vi "4155C Output-FPP Config SMUs v3.1.vi"(0 "VISA resource name in":refnum<visa-resource-name>, 1 "Pulse period":dbl=0.005 min=0.005 max=1.0 step=0.0001 format="%.4f", 2 "FPP - Source":u32(ring)=6 items=["SMU1  ", "SMU2  ", "SMU3  ", "SMU4  ", "SMU5  ", "SMU6  ", "VSU1  ", "VSU2  "], 3 "Pulse width":dbl=0.0005 min=0.0005 max=0.1 step=0.0001 format="%.4f", 4 "Base voltage":dbl format="%^.4e", 5 "error in (no error)":errorcluster, 6 "sweep method":u16(ring) items=["Continuous", "Pulsed"], 7 "FPP - Gate":u32(ring)=2 items=["SMU1  ", "SMU2  ", "SMU3  ", "SMU4  ", "SMU5  ", "SMU6  ", "VSU1  ", "VSU2  "], 8 "FPP - Drain":u32(ring)=1 items=["SMU1  ", "SMU2  ", "SMU3  ", "SMU4  ", "SMU5  ", "SMU6  ", "VSU1  ", "VSU2  "], 9 "FPP - Probe 1":u32(ring) items=["SMU1  ", "SMU2  ", "SMU3  ", "SMU4  ", "SMU5  ", "SMU6  ", "VSU1  ", "VSU2  "], 10 "Gate mode":u16(ring) items=["Auto", "Limited", "Fixed"], 11 "Source/drain mode":u16(ring) items=["Auto", "Limited", "Fixed"], 12 "Gate Range":u8(slide)=6 max=11 scale=0.0..11.0, 13 "Source/drain Range":u8(slide)=6 max=11 scale=0.0..11.0, 15 "FPP - Probe 2":u32(ring)=3 items=["SMU1  ", "SMU2  ", "SMU3  ", "SMU4  ", "SMU5  ", "SMU6  ", "VSU1  ", "VSU2  "]) -> (14 "VISA Resource Name out":refnum<visa-resource-name>, 19 "error out":errorcluster)   [LabVIEW 2016]
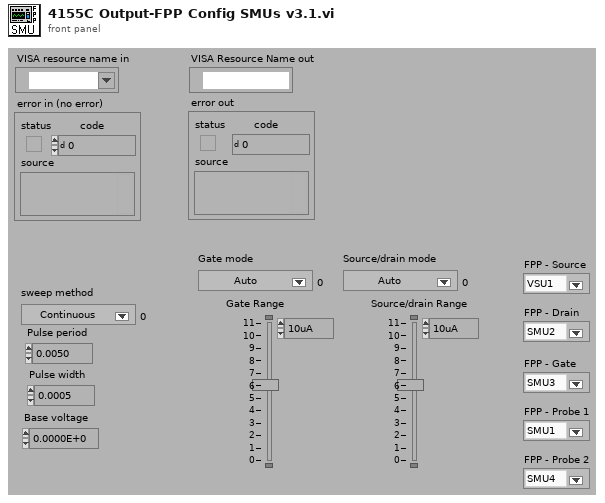
[diagram p1: front panel]
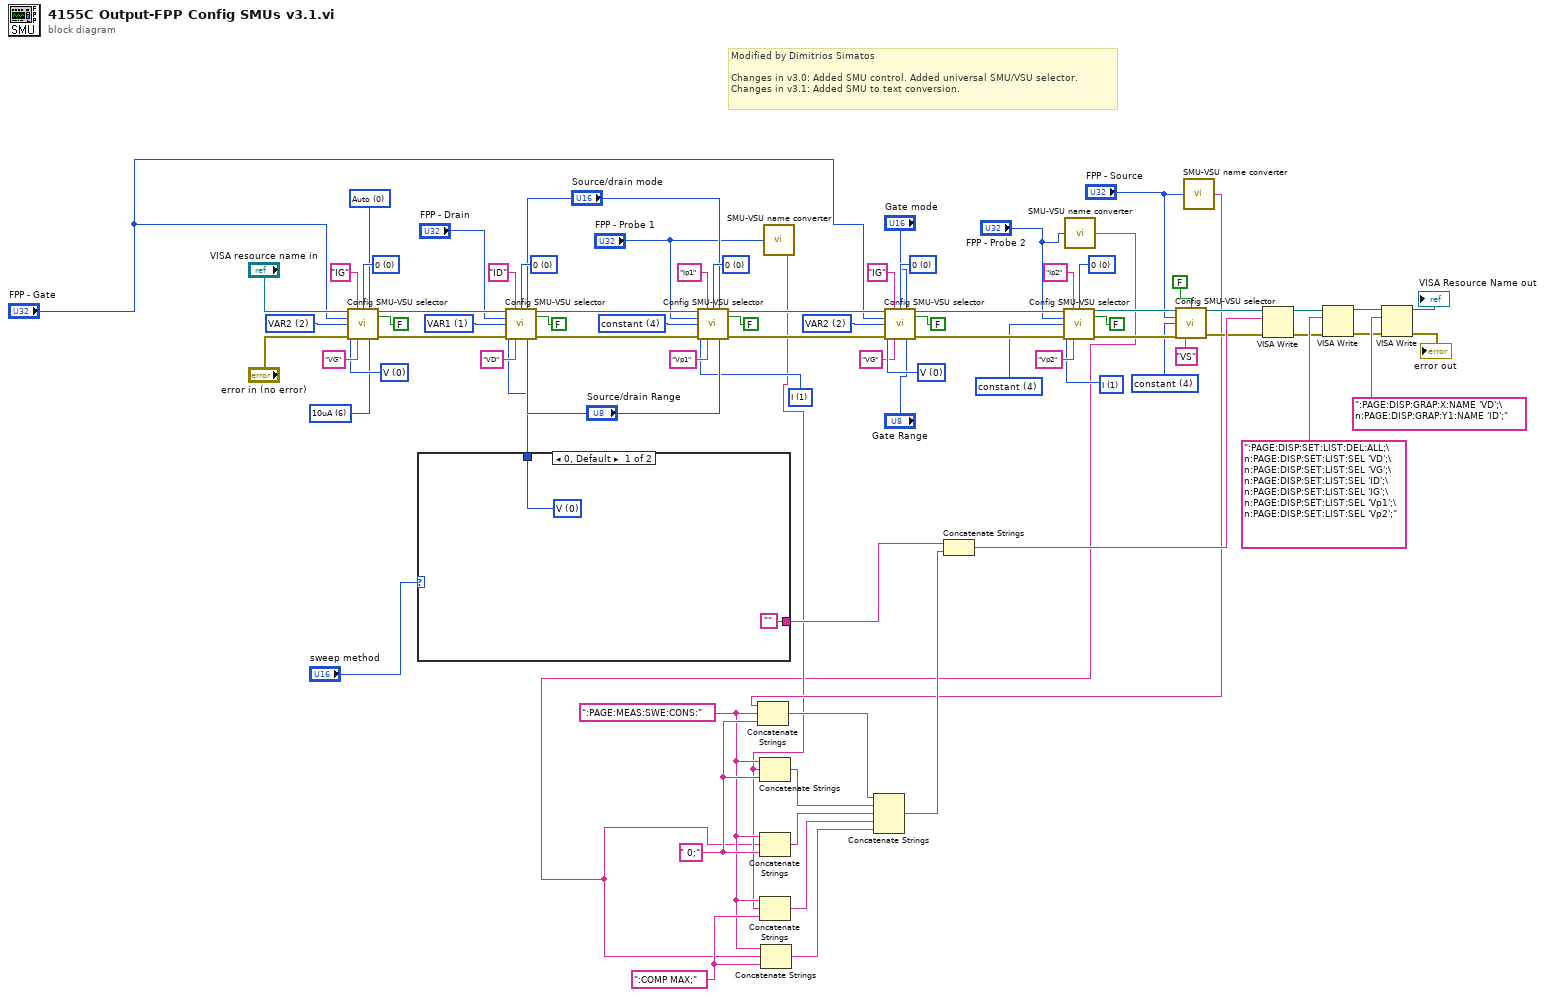
[diagram p0: block diagram]
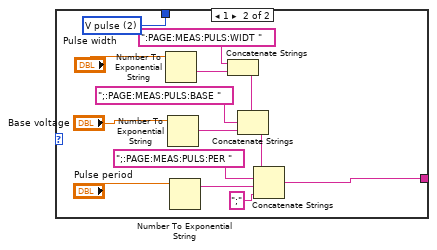
[diagram p2: hidden frame]
diagram:
  w11 = ":COMP MAX;" ("write buffer (\"\")")
  w13 = " 0;" ("write buffer (\"\")")
  w10 = ":PAGE:MEAS:SWE:CONS:" ("write buffer (\"\")")
  w30 = u32 4 items=["disabled  ", "VAR1  ", "VAR2  ", "VAR1'  ", "constant  "] ("function")
  w34 = u32 4 items=["disabled  ", "VAR1  ", "VAR2  ", "VAR1'  ", "constant  "] ("function")
  w36 = u32 1 items=["V  ", "I  ", "V pulse  ", "I pulse  ", "  common  "] ("mode")
  w37 = u16 0 items=["Auto", "Limited", "Fixed"] ("Range mode")
  w38 = u8 6 items=["10fA  ", "100fA  ", "1nA  ", "10nA", "100nA", "1uA", "10uA", "100uA", "1mA", "10mA", "100mA", "1A"] ("Range")
  w43 = u32 2 items=["disabled  ", "VAR1  ", "VAR2  ", "VAR1'  ", "constant  "] ("function")
  w45 = u32 0 items=["0  ", "10K Ohms  ", "100K Ohms  ", "1M Ohms  "] ("series resistance *")
  w46 = u32 0 items=["V  ", "I  ", "V pulse  ", "I pulse  ", "  common  "] ("mode")
  w64 = u32 0 items=["0  ", "10K Ohms  ", "100K Ohms  ", "1M Ohms  "] ("series resistance *")
  w68 = u32 0 items=["V  ", "I  ", "V pulse  ", "I pulse  ", "  common  "] ("mode")
  w69 = u32 0 items=["0  ", "10K Ohms  ", "100K Ohms  ", "1M Ohms  "] ("series resistance *")
  w71 = u32 2 items=["disabled  ", "VAR1  ", "VAR2  ", "VAR1'  ", "constant  "] ("function")
  w74 = u32 0 items=["0  ", "10K Ohms  ", "100K Ohms  ", "1M Ohms  "] ("series resistance *")
  w76 = u32 4 items=["disabled  ", "VAR1  ", "VAR2  ", "VAR1'  ", "constant  "] ("function")
  w50 = u32 1 items=["V  ", "I  ", "V pulse  ", "I pulse  ", "  common  "] ("mode")
  w79 = u32 0 items=["0  ", "10K Ohms  ", "100K Ohms  ", "1M Ohms  "] ("series resistance *")
  w81 = u32 1 items=["disabled  ", "VAR1  ", "VAR2  ", "VAR1'  ", "constant  "] ("function")
  # "Modified by Dimitrios Simatos\n\nChanges in v3.0: Added SMU control. Added universal SMU/VSU selector.\nChanges in v3.1: Added SMU to text conversion."
  n1 = call "Config SMU-VSU selector.vi"("VISA session"="VISA resource name in", "I name (max 6 chars)"="IG", "standby"=FALSE, "Range mode"=w37, "unit to configure"="FPP - Gate", "function"=w43, "mode"=w46, "error in (no error)"="error in (no error)", "V name (max 6 chars)"="VG", "series resistance *"=w45, "Range"=w38) -> ("dup VISA resource name"=w40:refnum<visa-resource-name>, "error out"=w41:errorcluster)  [unwired: 1 in, 2 out]
  n2 = case shown="0, Default" "sweep method" {
    tunnel: [w83 w97] -> w49
    tunnel: ["" w88] -> w35
    frame 0, Default {
      w83 = u32 0 items=["V  ", "I  ", "V pulse  ", "I pulse  ", "  common  "] ("mode")
    }
    frame 1 {
      w97 = u32 2 items=["V  ", "I  ", "V pulse  ", "I pulse  ", "  common  "] ("mode")
      n3 = Number To Exponential String(number="Pulse width") -> (E-format string=w96:string)  [unwired: 3 in]
      n4 = Number To Exponential String(number="Base voltage") -> (E-format string=w92:string)  [unwired: 3 in]
      n5 = Number To Exponential String(number="Pulse period") -> (E-format string=w89:string)  [unwired: 3 in]
      n6 = Concatenate Strings(":PAGE:MEAS:PULS:WIDT " ("Substring"), w96) -> (w94:string)
      n7 = Concatenate Strings(w94, ";:PAGE:MEAS:PULS:BASE " ("Substring"), w92) -> (w90:string)
      n8 = Concatenate Strings(w90, ";:PAGE:MEAS:PULS:PER " ("Substring"), w89, ";" ("Substring")) -> (w88:string)
    }
  }
  n9 = call "Config SMU-VSU selector.vi"("VISA session"=w40, "I name (max 6 chars)"="ID", "standby"=FALSE, "Range mode"="Source/drain mode", "unit to configure"="FPP - Drain", "function"=w81, "mode"=w49, "error in (no error)"=w41, "V name (max 6 chars)"="VD", "series resistance *"=w79, "Range"="Source/drain Range") -> ("dup VISA resource name"=w61:refnum<visa-resource-name>, "error out"=w60:errorcluster)  [unwired: 1 in, 2 out]
  n10 = call "Config SMU-VSU selector.vi"("VISA session"=w61, "I name (max 6 chars)"="Ip1", "standby"=FALSE, "Range mode"="Source/drain mode", "unit to configure"="FPP - Probe 1", "function"=w76, "mode"=w50, "error in (no error)"=w60, "V name (max 6 chars)"="Vp1", "series resistance *"=w74, "Range"="Source/drain Range") -> ("dup VISA resource name"=w58:refnum<visa-resource-name>, "error out"=w59:errorcluster)  [unwired: 1 in, 2 out]
  n11 = call "SMU-VSU name converter.vi"("unit to configure"="FPP - Probe 1") -> ("SMU/VSU to be configured"=w3:string)
  n12 = Concatenate Strings(w10, w3, w13) -> (w14:string)
  n13 = Concatenate Strings(w10, w3, w11) -> (w9:string)
  n14 = call "Config SMU-VSU selector.vi"("VISA session"=w58, "I name (max 6 chars)"="IG", "standby"=FALSE, "Range mode"="Gate mode", "unit to configure"="FPP - Gate", "function"=w71, "mode"=w68, "error in (no error)"=w59, "V name (max 6 chars)"="VG", "series resistance *"=w69, "Range"="Gate Range") -> ("dup VISA resource name"=w57:refnum<visa-resource-name>, "error out"=w56:errorcluster)  [unwired: 1 in, 2 out]
  n15 = call "Config SMU-VSU selector.vi"("VISA session"=w57, "I name (max 6 chars)"="Ip2", "standby"=FALSE, "unit to configure"="FPP - Probe 2", "function"=w34, "mode"=w36, "error in (no error)"=w56, "V name (max 6 chars)"="Vp2", "series resistance *"=w64) -> ("dup VISA resource name"=w32:refnum<visa-resource-name>, "error out"=w33:errorcluster)  [unwired: 3 in, 2 out]
  n16 = call "SMU-VSU name converter.vi"("unit to configure"="FPP - Probe 2") -> ("SMU/VSU to be configured"=w1:string)
  n17 = Concatenate Strings(w10, w1, w13) -> (w12:string)
  n18 = Concatenate Strings(w10, w1, w11) -> (w8:string)
  n19 = call "Config SMU-VSU selector.vi"("VISA session"=w32, "standby"=FALSE, "unit to configure"="FPP - Source", "function"=w30, "error in (no error)"=w33, "V name (max 6 chars)"="VS") -> ("dup VISA resource name"=w24:refnum<visa-resource-name>, "error out"=w19:errorcluster)  [unwired: 6 in, 2 out]
  n20 = call "SMU-VSU name converter.vi"("unit to configure"="FPP - Source") -> ("SMU/VSU to be configured"=w4:string)
  n21 = Concatenate Strings(w4, w10, w13) -> (w15:string)
  n22 = Concatenate Strings(w15, w14, w12, w9, w8) -> (w7:string)
  n23 = Concatenate Strings(w35, w7) -> (w27:string)
  n24 = VISA Write(VISA resource name=w24, write buffer=w27, error in (no error)=w19) -> (VISA resource name out=w28:refnum<visa-resource-name>, error out=w18:errorcluster)  [unwired: 1 out]
  n25 = VISA Write(VISA resource name=w28, write buffer=":PAGE:DISP:SET:LIST:DEL:ALL;\n:PAGE:DISP:SET:LIST:SEL 'VD';\n:PAGE:DISP:SET:LIST:SEL 'VG';\n:PAGE:DISP:SET:LIST:SEL 'ID';\n:PAGE:DISP:SET:LIST:SEL 'IG';\n:PAGE:DISP:SET:LIST:SEL 'Vp1';\n:PAGE:DISP:SET:LIST:SEL 'Vp2';" ("write buffer (\"\")"), error in (no error)=w18) -> (VISA resource name out=w23:refnum<visa-resource-name>, error out=w20:errorcluster)  [unwired: 1 out]
  n26 = VISA Write(VISA resource name=w23, write buffer=":PAGE:DISP:GRAP:X:NAME 'VD';\n:PAGE:DISP:GRAP:Y1:NAME 'ID';" ("write buffer (\"\")"), error in (no error)=w20) -> (VISA resource name out=→"VISA Resource Name out":refnum<visa-resource-name>, error out=→"error out":errorcluster)  [unwired: 1 out]
